vi "Clear Interlock Alarm.vi"(8 "error in (no error)":errorcluster, 11 "GEN40-38-LAN in":refnum<class "GEN40-38-LAN.lvclass">) -> (0 "error out":errorcluster, 3 "GEN40-38-LAN out":refnum<class "GEN40-38-LAN.lvclass">)   [LabVIEW 2018, in "GEN40-38-LAN.lvlib" / "GEN40-38-LAN.lvclass"]
uses:
  GEN40-38-LAN.lvclass
  PPLs/Power Supply/Parent/Power_Supply.lvlibp/Power Supply.lvclass
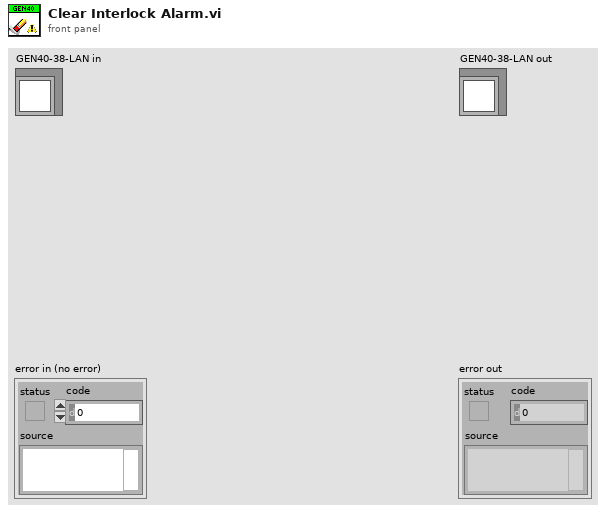
[diagram p1: front panel]
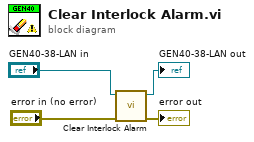
[diagram p0: block diagram]
diagram:
  n1 = call-parent "Clear Interlock Alarm.vi"("error in (no error)"="error in (no error)", "Power Supply in"="GEN40-38-LAN in") -> ("error out"=→"error out":errorcluster, "Power Supply out"=→"GEN40-38-LAN out":refnum<class "GEN40-38-LAN.lvclass">)  [unwired: 8 in]
